vi "Calculator-setup.vi"(7 "test case ID":string) -> (0 "error in (no error)":errorcluster, 1 "Operation":T1, 2 "b":dbl, 3 "a":dbl)   [LabVIEW 2015]
uses:
  Operation.ctl
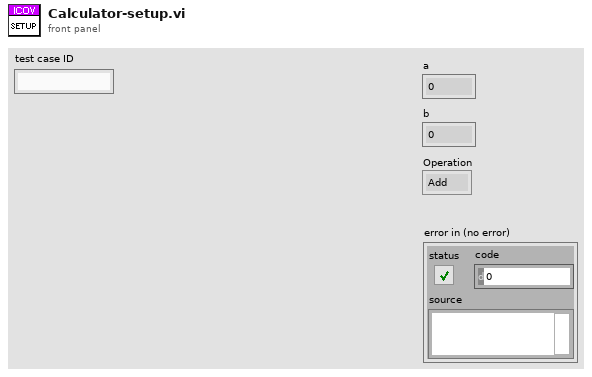
[diagram p1: front panel]
types:
  T1 = typedef "Operation.ctl" = enum16{"Add", "Subtract", "Multiply", "Divide"}
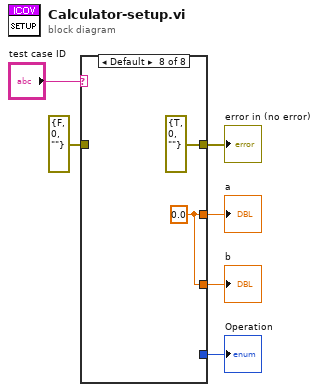
[diagram p0: block diagram]
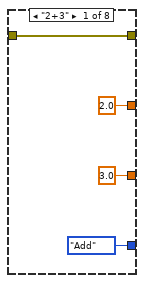
[diagram p2: hidden frame]
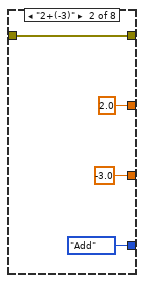
[diagram p3: hidden frame]
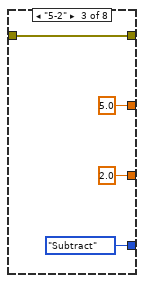
[diagram p4: hidden frame]
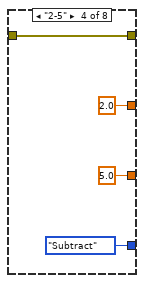
[diagram p5: hidden frame]
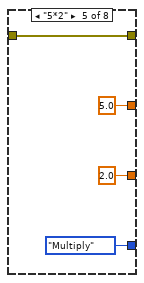
[diagram p6: hidden frame]
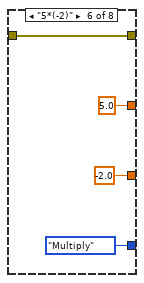
[diagram p7: hidden frame]
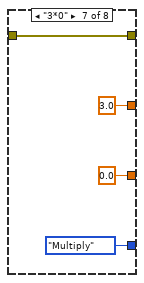
[diagram p8: hidden frame]
diagram:
  n1 = case shown="Default" "test case ID" {
    tunnel: [2.0 2.0 5.0 2.0 5.0 5.0 3.0 w35] -> w5
    tunnel: [3.0 -3.0 2.0 5.0 2.0 -2.0 0.0 w35] -> w4
    tunnel: [w8 w11 w18 w22 w26 w30 w34 errorcluster {"status"=TRUE, "code"=0, "source"=""} ("error in (no error)")] -> w3
    tunnel: errorcluster {"status"=FALSE, "code"=0, "source"=""} ("error in (no error)") -> [w8 w11 w18 w22 w26 w30 w34 _]
    tunnel: [Operation."Add" ("Operation") Operation."Add" ("Operation") Operation."Subtract" ("Operation") Operation."Subtract" ("Operation") Operation."Multiply" ("Operation") Operation."Multiply" ("Operation") Operation."Multiply" ("Operation") _] -> w1
    frame "2+3" {
    }
    frame "2+(-3)" {
    }
    frame "5-2" {
    }
    frame "2-5" {
    }
    frame "5*2" {
    }
    frame "5*(-2)" {
    }
    frame "3*0" {
    }
    frame Default {
      w35 = 0.0
    }
  }
  "a" <- w5
  "b" <- w4
  "Operation" <- w1
  "error in (no error)" <- w3
